vi "Drive Controller.vi"(8 "error in":errorcluster) -> ()   [LabVIEW 2019]
doc: "This VI executes continuously carrying out the current operation and responding to updates or new operation requests. It will often contain the timing or control code that is difficult to place directly in TeleOp. This VI generally opens all sensors and motors and isolates the rest of the robot code from knowing implementation details of how the operations are carried out."
uses:
  <vilib>/Rock Robotics/WPI/Framework/Completion Status.ctl
  Drive Setpoints.ctl
  Drive Operations.ctl
  <vilib>/Rock Robotics/WPI/ThirdParty/Phoenix-LabVIEW/Motor Controller/Controls/CTRE_Phoenix_MotorControl_ControlMode.ctl
  <vilib>/Rock Robotics/WPI/ThirdParty/Phoenix-LabVIEW/Motor Controller/Get/CTRE_Phoenix_MotorController_GetQuadratureData.vi
  <vilib>/Rock Robotics/WPI/SafetyOutput/WPI_SafetyOutputConfigMenu.ctl
  <vilib>/Rock Robotics/WPI/ThirdParty/Phoenix-LabVIEW/Motor Controller/Get/CTRE_Phoenix_MotorController_GetSelectedSensorData.vi
  <vilib>/Rock Robotics/WPI/RobotDrive/WPI_RobotDriveOpen2MotorWithExistingMotors.vi
panel:
  out "Iterations":i32
  out "Analog Position":dbl
  in  "Interactive Values":T1
  in  "Buttons":cluster{"Execute Cmd":bool, "Abort Cmd":bool}
  out "Command Timing":cluster{"Start Time (ms)":u32, "Iterations":i32}
  out "Status":T3
  out "Current\nCmd":string
  # "Tip: The graph shows the motor setpoints. It may also be helpful to observe inputs and sensor values.\nYou may also want to display tuning or debugging controls."
  # "Interactive Command: You may fill in the settings for a command\nand schedule it with the Execute button. You can observe and abort\nany command while fine tuning the code for the controller."
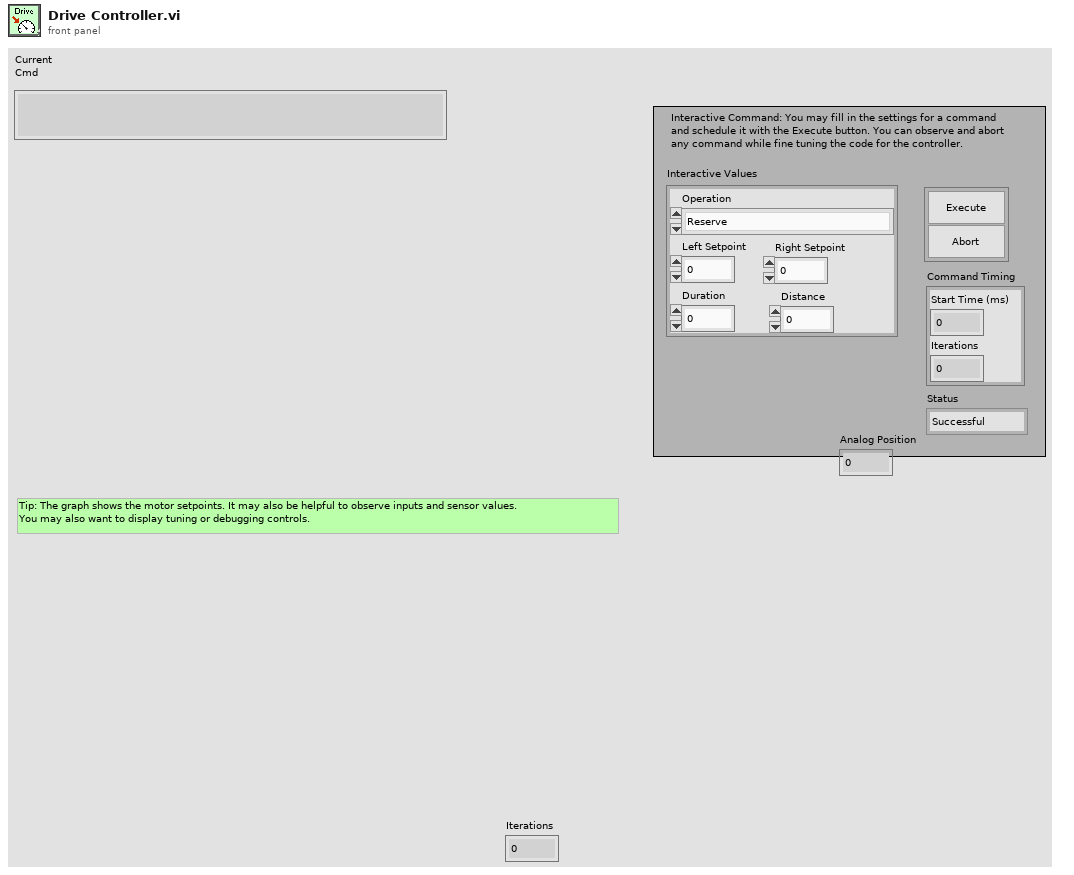
[diagram p1: front panel]
types:
  T1 = typedef "Drive Setpoints.ctl" = cluster{"Operation":T2, "Left Setpoint":dbl, "Right Setpoint":dbl, "Duration":dbl, "Distance":dbl}
  T2 = typedef "Drive Operations.ctl" = enum16{"Reserve", "Read Current", "Immediate", "Drive for Time", "Drive for Distance", "Turn angle"}
  T3 = typedef "Completion Status.ctl" = enum16{"Successful", "Aborted", "Incomplete"}
  T4 = typedef "WPI_SafetyOutputConfigMenu.ctl" = enum16{"Enable", "Disable"}
  T5 = typedef "WPI_MotorControlDeviceRef.ctl" = cluster{"DeviceStatus":errorcluster, "Type":T6, "PWM":cluster{"PWM Channel":T7, "DeadBand":T8}, "CAN":cluster{"Device Number":u8, "SetOutput VI Ref":variant, "GetOutput VI Ref":variant, "Enable VI Ref":variant, "Disable VI Ref":variant, "Data":variant}, "Invert":bool, "DIO PWM":cluster{"PWM \"Enable\" Channel":T7, "DIOChannel":T9, "PWM Rate":dbl}}
  T6 = typedef "WPI_MotorControlType.ctl" = enum16{"PWM", "CAN", "DIO PWM"}
  T7 = typedef "FPGA_DIOPWMChannel.ctl" = enum8{"PWM 0", "PWM 1", "PWM 2", "PWM 3", "PWM 4", "PWM 5", "PWM 6", "PWM 7", "PWM 8", "PWM 9", "PWM MXP 0", "PWM MXP 1", "PWM MXP 2", "PWM MXP 3", "PWM MXP 4", "PWM MXP 5", "PWM MXP 6", "PWM MXP 7", "PWM MXP 8", "PWM MXP 9", "Invalid"}
  T8 = typedef "WPI_PWMDeadband.ctl" = cluster{"Name":string, "maxPositivePwm":i32, "minPositivePwm":i32, "centerPwm":i32, "maxNegativePwm":i32, "minNegativePwm":i32, "angularRange":u16}
  T9 = typedef "FPGA_DIOChannel.ctl" = enum8{"DIO 0", "DIO 1", "DIO 2", "DIO 3", "DIO 4", "DIO 5", "DIO 6", "DIO 7", "DIO 8", "DIO 9", "DIO MXP 0", "DIO MXP 1", "DIO MXP 2", "DIO MXP 3", "DIO MXP 4", "DIO MXP 5", "DIO MXP 6", "DIO MXP 7", "DIO MXP 8", "DIO MXP 9", "DIO MXP 10", "DIO MXP 11", "DIO MXP 12", "DIO MXP 13", "DIO MXP 14", "DIO MXP 15", "SPI Port CS1", "SPI Port CS2", "SPI Port CS3", "SPI Port MISO", "SPI Port MOSI", "Invalid"}
  T10 = typedef "WPI_RobotDriveDevRef.ctl" = cluster{"DevStatus":errorcluster, "Motors[]":T5[], "Square Inputs":bool, "Max Output":dbl}
  T11 = enum16{"FollowerType_PercentOutput", "FollowerType_AuxOutput1"}
  T12 = typedef "Command Status Info.ctl" = cluster{"Name":string, "Status":T3, "notifier out":T13}
  T13 = typedef "Completion Notifier.ctl" = refnum<notifier>
  T14 = cluster{"SubSystem Data":T1, cluster{"Start Time (ms)":u32, "Iterations":i32}, cluster{"Command Info":T12, "Description":string, "Default Command":T1, "queue out":refnum<queue>, "Subsystem Name":string}}
  T15 = typedef "CTRE_Phoenix_MotorControl_ControlMode.ctl" = u16
  T16 = cluster{"SubSystem Data":T1, cluster{"Start Time (ms)":u32, "Iterations":i32}, "Default Command Arguments":cluster{"Command Info":T12, "Description":string, "Default Command":T1, "queue out":refnum<queue>, "Subsystem Name":string}}
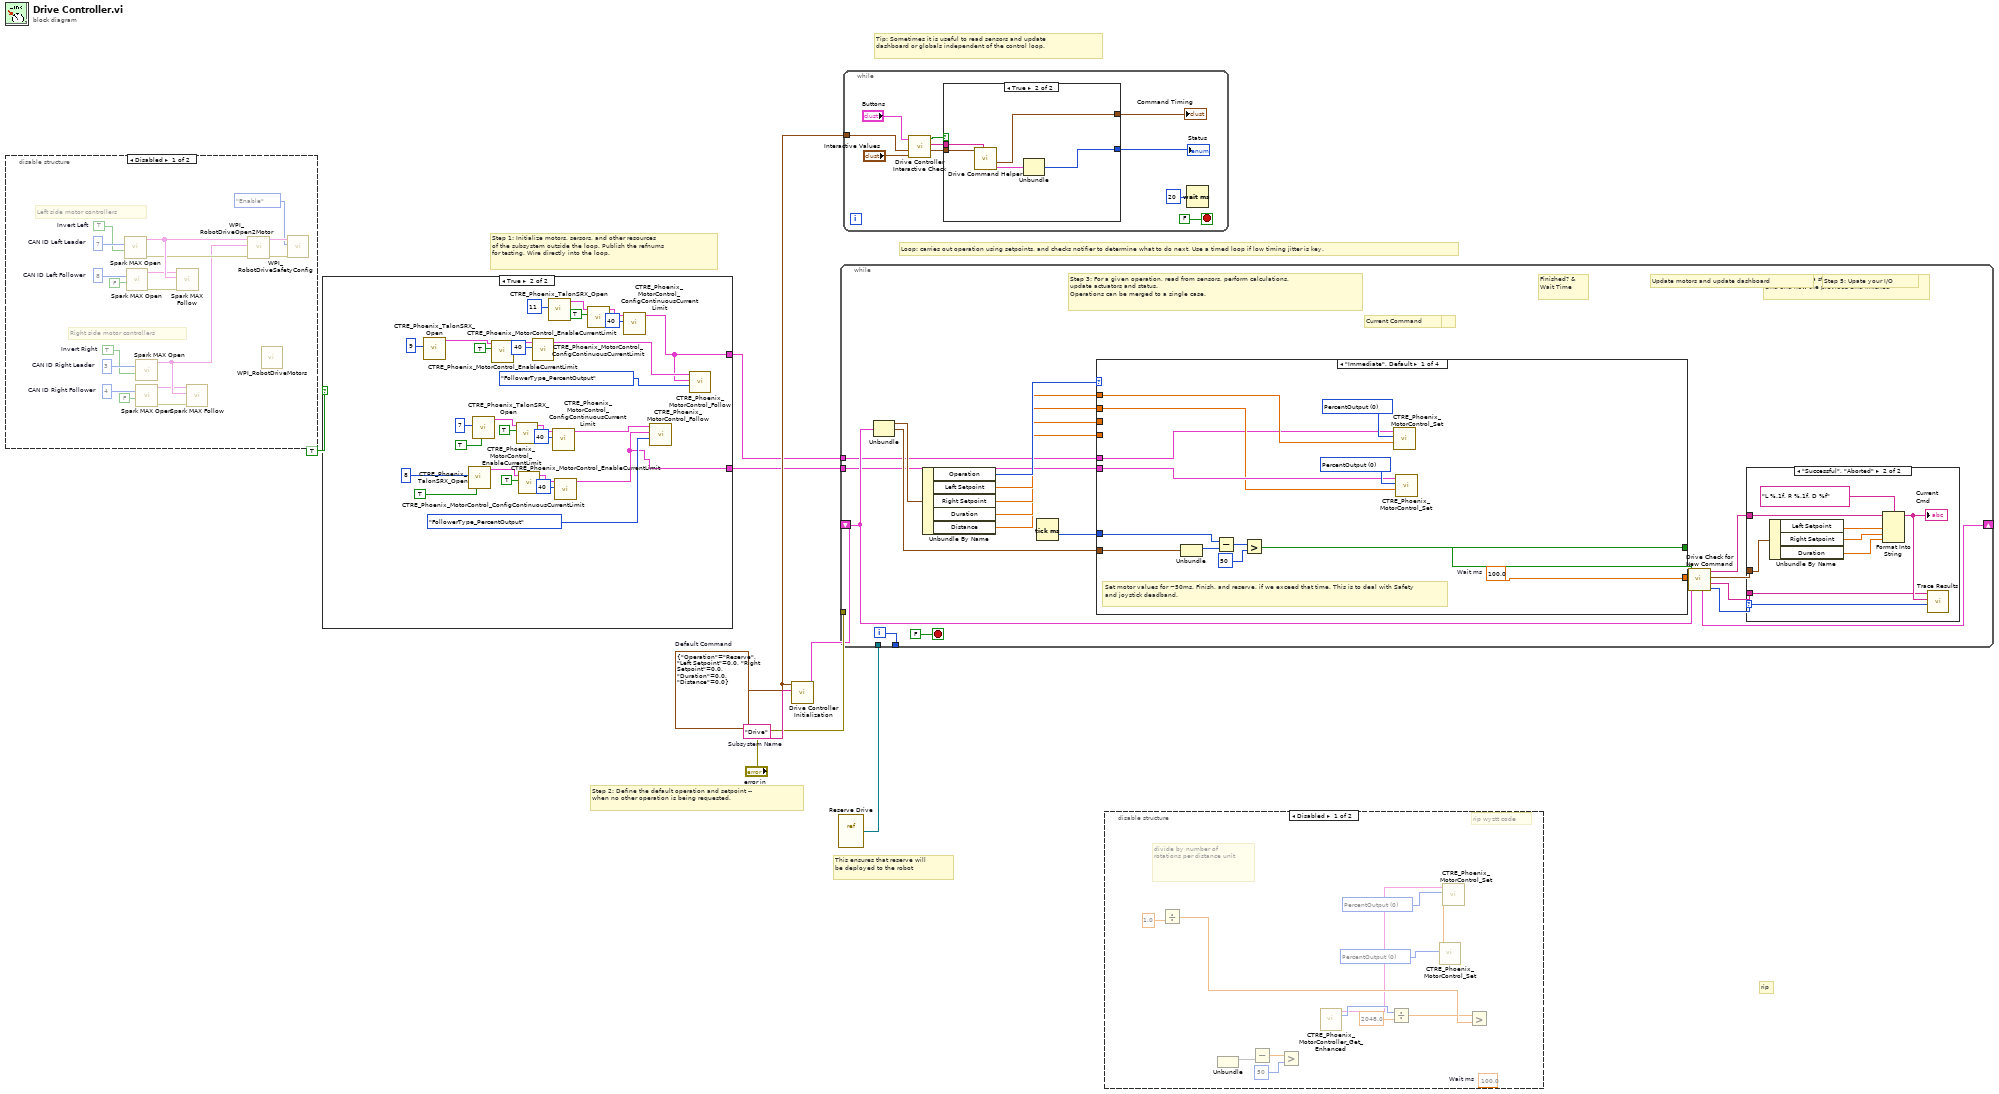
[diagram p0: block diagram]
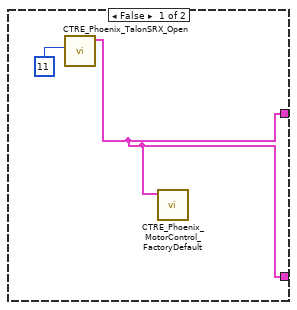
[diagram p2: hidden frame]
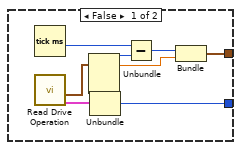
[diagram p5: hidden frame]
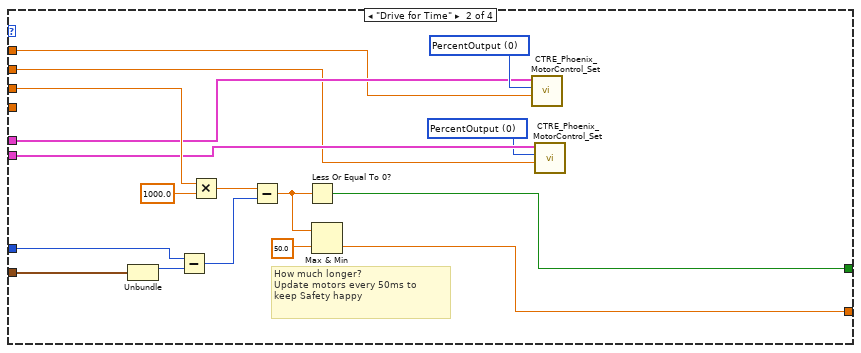
[diagram p7: hidden frame]
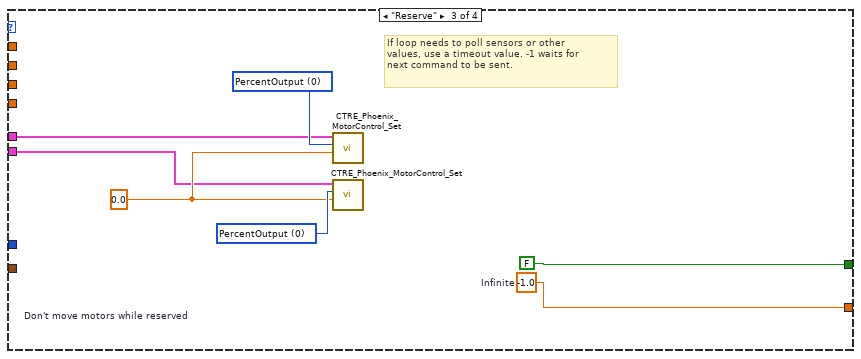
[diagram p8: hidden frame]
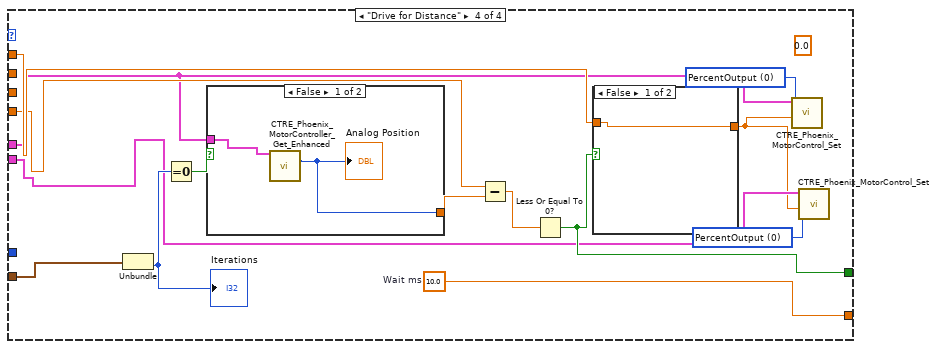
[diagram p9: hidden frame]
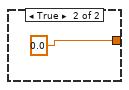
[diagram p10: hidden frame]
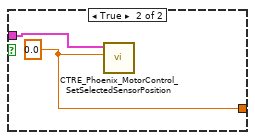
[diagram p11: hidden frame]
diagram:
  w4 = T1 {"Operation"=enum."Reserve", "Left Setpoint"=0.0, "Right Setpoint"=0.0, "Duration"=0.0, "Distance"=0.0}  # Default Command
  w8 = "Drive"  # Subsystem Name
  # "rip"
  # "This ensures that reserve will\nbe deployed to the robot"
  # "Tip: Sometimes it is useful to read sensors and update\ndashboard or globals independent of the control loop."
  # "Step 2: Define the default operation and setpoint --\nwhen no other operation is being requested."
  # "Step 1: Initialize motors, sersors, and other resources\nof the subsystem outside the loop. Publish the refnums\nfor testing. Wire directly into the loop."
  # "Loop: carries out operation using setpoints, and checks notifier to determine what to do next. Use a timed loop if low timing jitter is key."
  n1 = disable-structure shown="Disabled" {
    frame Disabled {
      w15 = TRUE  # Invert Left
      w14 = TRUE  # Invert Right
      w20 = u8 3  # CAN ID Right Leader
      w19 = u8 4  # CAN ID Right Follower
      w26 = u8 7  # CAN ID Left Leader
      w27 = u8 8  # CAN ID Left Follower
      # "Right side motor controllers"
      # "Left side motor controllers"
      n2 = call <vilib>:"Spark MAX Open.vi"("Invert"=w15, "Device Number"=w26) -> ("error out"=w24:errorcluster, "MotorControlDeviceRef"=w25:T5)  [unwired: 8 in]
      n3 = call <vilib>:"Spark MAX Open.vi"("Invert"=FALSE, "Device Number"=w27) -> ("error out"=w22:errorcluster, "MotorControlDeviceRef"=w23:T5)  [unwired: 8 in]
      n4 = call <vilib>:"Spark MAX Open.vi"("Invert"=w14, "Device Number"=w20) -> ("MotorControlDeviceRef"=w11:T5)  [unwired: 8 in, 1 out]
      n5 = call <vilib>:"Spark MAX Open.vi"("Invert"=FALSE, "Device Number"=w19) -> ("error out"=w21:errorcluster, "MotorControlDeviceRef"=w9:T5)  [unwired: 8 in]
      n6 = call <vilib>:"Spark MAX Follow.vi"("error in (no error)"=w22, "Master Controller"=w25, "MotorControlDeviceRef"=w23) -> ()  [unwired: 7 in, 2 out]
      n7 = call <vilib>:"Spark MAX Follow.vi"("error in (no error)"=w21, "Master Controller"=w11, "MotorControlDeviceRef"=w9) -> ()  [unwired: 7 in, 2 out]
      n8 = call-poly <vilib>:"WPI_RobotDriveOpen2Motor.vi"("error in (no error)"=w24, "Right Motor Dev Ref"=w11, "Left Motor Dev Ref"=w25) -> ("error out"=w17:errorcluster, "RobotDriveDevRef"=w18:T10)  [unwired: 7 in]
      n9 = call <vilib>:"WPI_RobotDriveMotors.vi"() -> ()  [unwired: 4 in, 8 out]
      n10 = call <vilib>:"WPI_RobotDriveSafetyConfig.vi"("error in (no error)"=w17, "mode"=WPI_SafetyOutputConfigMenu."Enable", "RobotDriveDevRef"=w18) -> ("RobotDriveDevRef"=w10:T10)  [unwired: 7 in, 1 out]
    }
    frame Enabled {
    }
  }
  n11 = case shown="True" TRUE {
    tunnel: [w28 w34] -> w3
    tunnel: [w28 w46] -> w2
    frame False {
      n12 = call <vilib>:"CTRE_Phoenix_TalonSRX_Open.vi"("Device Number"=u8 11) -> ("CAN Talon SRX Ref"=w28:T5)  [unwired: 9 in, 1 out]
      n13 = call <vilib>:"CTRE_Phoenix_MotorControl_FactoryDefault.vi"("PhoenixMotorControlDevRef"=w28) -> ()  [unwired: 9 in, 2 out]
    }
    frame True {
      n14 = call <vilib>:"CTRE_Phoenix_TalonSRX_Open.vi"("Device Number"=u8 9) -> ("CAN Talon SRX Ref"=w39:T5)  [unwired: 9 in, 1 out]
      n15 = call <vilib>:"CTRE_Phoenix_TalonSRX_Open.vi"("Invert"=TRUE, "Device Number"=u8 8) -> ("CAN Talon SRX Ref"=w48:T5)  [unwired: 8 in, 1 out]
      n16 = call <vilib>:"CTRE_Phoenix_TalonSRX_Open.vi"("Invert"=TRUE, "Device Number"=u8 7) -> ("CAN Talon SRX Ref"=w43:T5)  [unwired: 8 in, 1 out]
      n17 = call <vilib>:"CTRE_Phoenix_MotorControl_EnableCurrentLimit.vi"("Enable Current Limit?"=TRUE, "PhoenixMotorControlDevRef"=w39) -> ("PhoenixMotorControlDevRef"=w40:T5)  [unwired: 8 in, 1 out]
      n18 = call <vilib>:"CTRE_Phoenix_MotorControl_EnableCurrentLimit.vi"("Enable Current Limit?"=TRUE, "PhoenixMotorControlDevRef"=w43) -> ("PhoenixMotorControlDevRef"=w44:T5)  [unwired: 8 in, 1 out]
      n19 = call <vilib>:"CTRE_Phoenix_MotorControl_EnableCurrentLimit.vi"("Enable Current Limit?"=TRUE, "PhoenixMotorControlDevRef"=w48) -> ("PhoenixMotorControlDevRef"=w47:T5)  [unwired: 8 in, 1 out]
      n20 = call <vilib>:"CTRE_Phoenix_MotorControl_ConfigContinuousCurrentLimit.vi"("Continuous Current Limit (Amps)"=40, "PhoenixMotorControlDevRef"=w40) -> ("PhoenixMotorControlDevRef"=w38:T5)  [unwired: 8 in, 1 out]
      n21 = call <vilib>:"CTRE_Phoenix_TalonSRX_Open.vi"("Device Number"=u8 11) -> ("CAN Talon SRX Ref"=w35:T5)  [unwired: 9 in, 1 out]
      n22 = call <vilib>:"CTRE_Phoenix_MotorControl_ConfigContinuousCurrentLimit.vi"("Continuous Current Limit (Amps)"=40, "PhoenixMotorControlDevRef"=w44) -> ("PhoenixMotorControlDevRef"=w42:T5)  [unwired: 8 in, 1 out]
      n23 = call <vilib>:"CTRE_Phoenix_MotorControl_ConfigContinuousCurrentLimit.vi"("Continuous Current Limit (Amps)"=40, "PhoenixMotorControlDevRef"=w47) -> ("PhoenixMotorControlDevRef"=w46:T5)  [unwired: 8 in, 1 out]
      n24 = call <vilib>:"CTRE_Phoenix_MotorControl_EnableCurrentLimit.vi"("Enable Current Limit?"=TRUE, "PhoenixMotorControlDevRef"=w35) -> ("PhoenixMotorControlDevRef"=w36:T5)  [unwired: 8 in, 1 out]
      n25 = call <vilib>:"CTRE_Phoenix_MotorControl_ConfigContinuousCurrentLimit.vi"("Continuous Current Limit (Amps)"=40, "PhoenixMotorControlDevRef"=w36) -> ("PhoenixMotorControlDevRef"=w34:T5)  [unwired: 8 in, 1 out]
      n26 = call <vilib>:"CTRE_Phoenix_MotorControl_Follow.vi"("FollowerType"=T11."FollowerType_PercentOutput", "Master Controller to Follow"=w46, "PhoenixMotorControlDevRef"=w42) -> ()  [unwired: 7 in, 2 out]
      n27 = call <vilib>:"CTRE_Phoenix_MotorControl_Follow.vi"("FollowerType"=T11."FollowerType_PercentOutput", "Master Controller to Follow"=w34, "PhoenixMotorControlDevRef"=w38) -> ()  [unwired: 7 in, 2 out]
    }
  }
  n28 = call "Drive Controller Initialization.vi"("Subsystem Name"=w8, "Default Command"=w4) -> ("Current Command"=w6:T14)  [unwired: 9 in]
  n29 = vi-ref "Reserve Drive.vi"() -> (w5:refnum<vi>)
  n30 = while {
    shift-right: [w68] -> _
    shift-left: w6 -> [w61]
    tunnel: [w76] -> _
    tunnel: "error in" -> [_]
    tunnel: w5 -> [_]
    tunnel: w2 -> [w59]
    tunnel: w3 -> [w58]
    i -> [w76]
    stop <- FALSE stop-if-true
    # "Step 5: Upate your I/O"
    # "Step 4: Format a string to describe this\ncmd and how the previous cmd finished"
    # "Current Command"
    # "Update motors and update dashboard"
    # "Access Cmd setpoints"
    # "Finished? &\nWait Time"
    # "Step 3: For a given operation, read from sensors, perform calculations,\nupdate actuators and status.\nOperations can be merged to a single case."
    n31 = Unbundle(w61) -> ("SubSystem Data"=w75:T1, w62:cluster{"Start Time (ms)":u32, "Iterations":i32})  [unwired: 1 out]
    n32 = Unbundle By Name(w75) -> ("Operation"=w74:T2, "Left Setpoint"=w73:dbl, "Right Setpoint"=w72:dbl, "Duration"=w71:dbl, "Distance"=w60:dbl)
    n33 = Tick Count (ms)() -> (millisecond timer value=w70:u32)
    n34 = case shown="\"Immediate\", Default" w74 {
      tunnel: [w99 w106 w123 w130] -> w67
      tunnel: [w94 w111 FALSE ("ignore previous (F)") w129] -> w66
      tunnel: w62 -> [w93 w113 _ w131]
      tunnel: w73 -> [w89 w102 _ w133]
      tunnel: w72 -> [w88 w101 _ _]
      tunnel: w71 -> [_ w110 _ _]
      tunnel: w70 -> [w95 w109 _ _]
      tunnel: w60 -> [_ _ _ w132]
      tunnel: w59 -> [w90 w103 w117 w128]
      tunnel: w58 -> [w87 w104 w118 w124]
      frame "Immediate", Default {
        w91 = T15 0 items=["PercentOutput"=0, "Position"=1, "Velocity"=2, "Current"=3, "Follower"=5, "MotionProfile"=6, "MotionMagic"=7, "MotionProfileArc"=10, "Disabled"=15] ("Control Mode")
        w92 = T15 0 items=["PercentOutput"=0, "Position"=1, "Velocity"=2, "Current"=3, "Follower"=5, "MotionProfile"=6, "MotionMagic"=7, "MotionProfileArc"=10, "Disabled"=15] ("Control Mode")
        w99 = 100.0  # Wait ms
        # "Set motor values for ~50ms. Finish, and reserve, if we exceed that time. This is to deal with Safety and joystick deadband."
        n35 = Unbundle(w93) -> ("Start Time (ms)"=w96:u32)  [unwired: 1 out]
        n36 = Subtract(x=w95, y=w96) -> (x-y=w97:u32)
        n37 = Greater?(x=w97, y=u8 50 ("Left Motor")) -> (0:w94:bool)
        n38 = call <vilib>:"CTRE_Phoenix_MotorControl_Set.vi"("Output"=w89, "Control Mode"=w92, "PhoenixMotorControlDevRef"=w87) -> ()  [unwired: 7 in, 2 out]
        n39 = call <vilib>:"CTRE_Phoenix_MotorControl_Set.vi"("Output"=w88, "Control Mode"=w91, "PhoenixMotorControlDevRef"=w90) -> ()  [unwired: 7 in, 2 out]
      }
      frame "Drive for Time" {
        w100 = T15 0 items=["PercentOutput"=0, "Position"=1, "Velocity"=2, "Current"=3, "Follower"=5, "MotionProfile"=6, "MotionMagic"=7, "MotionProfileArc"=10, "Disabled"=15] ("Control Mode")
        w105 = T15 0 items=["PercentOutput"=0, "Position"=1, "Velocity"=2, "Current"=3, "Follower"=5, "MotionProfile"=6, "MotionMagic"=7, "MotionProfileArc"=10, "Disabled"=15] ("Control Mode")
        # "How much longer?\nUpdate motors every 50ms to\nkeep Safety happy"
        n40 = Unbundle(w113) -> ("Start Time (ms)"=w112:u32)  [unwired: 1 out]
        n41 = Subtract(x=w109, y=w112) -> (x-y=w116:u32)
        n42 = Multiply(x=w110, y=1000.0) -> (x*y=w115:dbl)
        n43 = Subtract(x=w115, y=w116) -> (x-y=w108:dbl)
        n44 = Less Or Equal To 0?(x=w108) -> (x <= 0?=w111:bool)
        n45 = Max & Min(x=w108, y=50.0) -> (min(x,y)=w106:dbl)  [unwired: 1 out]
        n46 = call <vilib>:"CTRE_Phoenix_MotorControl_Set.vi"("Output"=w102, "Control Mode"=w105, "PhoenixMotorControlDevRef"=w104) -> ()  [unwired: 7 in, 2 out]
        n47 = call <vilib>:"CTRE_Phoenix_MotorControl_Set.vi"("Output"=w101, "Control Mode"=w100, "PhoenixMotorControlDevRef"=w103) -> ()  [unwired: 7 in, 2 out]
      }
      frame "Reserve" {
        w120 = T15 0 items=["PercentOutput"=0, "Position"=1, "Velocity"=2, "Current"=3, "Follower"=5, "MotionProfile"=6, "MotionMagic"=7, "MotionProfileArc"=10, "Disabled"=15] ("Control Mode")
        w121 = T15 0 items=["PercentOutput"=0, "Position"=1, "Velocity"=2, "Current"=3, "Follower"=5, "MotionProfile"=6, "MotionMagic"=7, "MotionProfileArc"=10, "Disabled"=15] ("Control Mode")
        w119 = 0.0  # Don't move motors while reserved
        w123 = -1.0  # Infinite
        # "If loop needs to poll sensors or other\nvalues, use a timeout value. -1 waits for\nnext command to be sent."
        n48 = call <vilib>:"CTRE_Phoenix_MotorControl_Set.vi"("Output"=w119, "Control Mode"=w121, "PhoenixMotorControlDevRef"=w118) -> ()  [unwired: 7 in, 2 out]
        n49 = call <vilib>:"CTRE_Phoenix_MotorControl_Set.vi"("Output"=w119, "Control Mode"=w120, "PhoenixMotorControlDevRef"=w117) -> ()  [unwired: 7 in, 2 out]
      }
      frame "Drive for Distance" {
        w125 = T15 0 items=["PercentOutput"=0, "Position"=1, "Velocity"=2, "Current"=3, "Follower"=5, "MotionProfile"=6, "MotionMagic"=7, "MotionProfileArc"=10, "Disabled"=15] ("Control Mode")
        w126 = T15 0 items=["PercentOutput"=0, "Position"=1, "Velocity"=2, "Current"=3, "Follower"=5, "MotionProfile"=6, "MotionMagic"=7, "MotionProfileArc"=10, "Disabled"=15] ("Control Mode")
        (unwired) 0.0 ("f")
        w130 = 10.0  # Wait ms
        n50 = Unbundle(w131) -> ("Iterations"=w137:i32)  [unwired: 1 out]
        "Iterations" <- w137
        n51 = Equal To 0?(x=w137) -> (x = 0?=w136:bool)
        n52 = case shown="False" w136 {
          tunnel: w124 -> [w141 w143]
          tunnel: [w140 w142] -> w135
          frame False {
            n53 = call-poly <vilib>:"CTRE_Phoenix_MotorController_Get_Enhanced.vi"("PhoenixMotorControlDevRef"=w141) -> ("Quadrature Position"=w140:i32)  [unwired: 11 in, 3 out]
            "Analog Position" <- w140
          }
          frame True {
            w142 = 0.0 ("Position")
            n54 = call <vilib>:"CTRE_Phoenix_MotorControl_SetSelectedSensorPosition.vi"("New Sensor Position"=w142, "PhoenixMotorControlDevRef"=w143) -> ()  [unwired: 8 in, 2 out]
          }
        }
        n55 = Subtract(x=w132, y=w135) -> (x-y=w134:dbl)
        n56 = Less Or Equal To 0?(x=w134) -> (x <= 0?=w129:bool)
        n57 = case shown="False" w129 {
          tunnel: [w138 0.0 ("Setpoint")] -> w127
          tunnel: w133 -> [w138 _]
          frame False {
          }
          frame True {
          }
        }
        n58 = call <vilib>:"CTRE_Phoenix_MotorControl_Set.vi"("Output"=w127, "Control Mode"=w126, "PhoenixMotorControlDevRef"=w124) -> ()  [unwired: 7 in, 2 out]
        n59 = call <vilib>:"CTRE_Phoenix_MotorControl_Set.vi"("Output"=w127, "Control Mode"=w125, "PhoenixMotorControlDevRef"=w128) -> ()  [unwired: 7 in, 2 out]
      }
    }
    n60 = call "Drive Check for New Command.vi"("input cluster"=w61, "Wait time (ms)"=w67, "Finished?"=w66) -> ("Completion"=w69:T3, "Subsystem Name"=w63:string, "Current Command"=w64:T1, "Initial Trace String"=w65:string, "Next Command"=w68:T16)  [unwired: 4 in]
    n61 = case shown="\"Successful\", \"Aborted\"" w69 {
      selector: w69 -> [_ w86]
      tunnel: w65 -> [_ w81]
      tunnel: w64 -> [_ w82]
      tunnel: w63 -> [_ w78]
      frame "Incomplete", Default {
        # "Continuing current command"
      }
      frame "Successful", "Aborted" {
        # "Report and setup for next command"
        n62 = Unbundle By Name(w82) -> ("Left Setpoint"=w84:dbl, "Right Setpoint"=w85:dbl, "Duration"=w79:dbl)
        n63 = Format Into String(format string="L %.1f, R %.1f, D %f", initial string=w81, w84, w85, w79) -> (resulting string=w80:string)  [unwired: 1 in, 1 out]
        "Current\nCmd" <- w80
        n64 = call <vilib>:"Trace Results.vi"("Status of previous command"=w86, "Description"=w80, "Subsystem"=w78) -> ()  [unwired: 9 in]
      }
    }
  }
  n65 = while {
    tunnel: w4 -> [w145]
    stop <- FALSE stop-if-true
    n66 = call "Drive Controller Interactive Check.vi"("Interactive Command In"="Interactive Values", "Default Command"=w145, "Buttons"="Buttons") -> ("Interactive Command Out"=w147:T1, "Trace String"=w148:string, "Schedule"=w149:bool)  [unwired: 6 in]
    n67 = case shown="True" w149 {
      tunnel: [w158 w166] -> w150
      tunnel: [w157 w162] -> w151
      tunnel: w148 -> [_ w164]
      tunnel: w147 -> [_ w163]
      frame False {
        n68 = Tick Count (ms)() -> (millisecond timer value=w161:u32)
        n69 = call "Read Drive Operation.vi"() -> ("Command Info"=w155:T12, "SubSystem Data"=w154:T1)  [unwired: 9 in, 1 out]
        n70 = Unbundle(w154) -> ("Operation"=w159:T2, "Left Setpoint"=w156:dbl)  [unwired: 3 out]
        n71 = Unbundle(w155) -> ("Status"=w158:T3)  [unwired: 2 out]
        n72 = Subtract(x=w161, y=w159) -> (x-y=w160:u32)
        n73 = Bundle(w160, "Left Setpoint"=w156) -> (w157:cluster{u32, "Left Setpoint":dbl})  [unwired: 1 in]
      }
      frame True {
        n74 = call "Drive Command Helper.vi"("Description"=w164, "SubSystem Data"=w163) -> ("Command Info Out"=w165:T12, "Command Timing"=w162:cluster{"Start Time (ms)":u32, "Iterations":i32})  [unwired: 7 in, 1 out]
        n75 = Unbundle(w165) -> ("Status"=w166:T3)  [unwired: 2 out]
      }
    }
    "Status" <- w150
    "Command Timing" <- w151
    n76 = Wait (ms)(milliseconds to wait=u32 20) -> ()  [unwired: 1 out]
  }
  n77 = disable-structure shown="Disabled" {
    frame Disabled {
      w171 = T15 0 items=["PercentOutput"=0, "Position"=1, "Velocity"=2, "Current"=3, "Follower"=5, "MotionProfile"=6, "MotionMagic"=7, "MotionProfileArc"=10, "Disabled"=15] ("Control Mode")
      w174 = T15 0 items=["PercentOutput"=0, "Position"=1, "Velocity"=2, "Current"=3, "Follower"=5, "MotionProfile"=6, "MotionMagic"=7, "MotionProfileArc"=10, "Disabled"=15] ("Control Mode")
      w179 = 100.0  # Wait ms
      # "rip wyztt code"
      # "divide by number of rotations per distance unit"
      n78 = Divide(y=1.0) -> (x/y=w183:dbl)  [unwired: 1 in]
      n79 = Unbundle() -> (w178:cluster{"Start Time (ms)":u32, "Iterations":i32}, "Start Time (ms)"=w177)  [unwired: 1 out]
      n80 = Subtract(y=w177) -> (x=w176:dbl, x-y=w180:dbl)
      n81 = Greater?(x=w180, y=u8 50 ("Left Motor")) -> ()  [unwired: 1 out]
      n82 = call <vilib>:"CTRE_Phoenix_MotorControl_Set.vi"("Control Mode"=w171) -> ("Output"=w175:dbl, "PhoenixMotorControlDevRef"=w168:T5)  [unwired: 7 in, 2 out]
      n83 = call-poly <vilib>:"CTRE_Phoenix_MotorController_Get_Enhanced.vi"("PhoenixMotorControlDevRef"=w168) -> ("Position (Raw Sensor Units)"=w170:i32)  [unwired: 11 in, 3 out]
      n84 = Divide(x=w170, y=2048.0) -> (x/y=w173:dbl)
      n85 = call <vilib>:"CTRE_Phoenix_MotorControl_Set.vi"("Output"=w175, "Control Mode"=w174) -> ("PhoenixMotorControlDevRef"=w167:T5)  [unwired: 7 in, 2 out]
      n86 = Greater?(x=w173, y=w183) -> (0:w169:bool)
    }
    frame Enabled {
    }
  }
